vi "SetProtocolState.vi"(9 "state":string) -> ()   [LabVIEW 2018]
uses:
  <vilib>/addons/_JKI.lib/REST Client/classes/REST Client/REST Client.lvclass
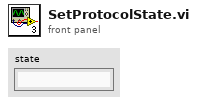
[diagram p1: front panel]
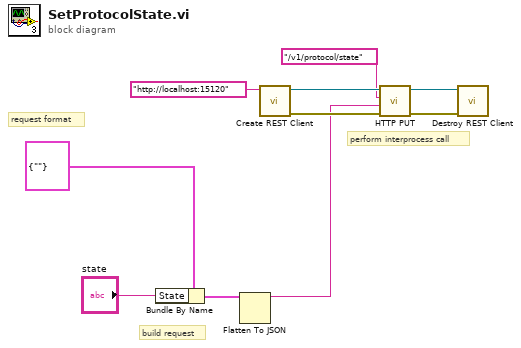
[diagram p0: block diagram]
diagram:
  # "build request"
  # "request format"
  # "perform interprocess call"
  n1 = Bundle By Name(cluster=cluster{"State":string} {"State"=""}, "State"="state") -> (w2:cluster{"State":string})
  n2 = Flatten To JSON(anything=w2) -> (JSON string=w4:string)  [unwired: 2 in, 1 out]
  n3 = call <vilib>:"Create REST Client.vi"("Base URL"="http://localhost:15120") -> ("error out"=w7:errorcluster, "REST Client out"=w9:refnum<class "REST Client.lvclass">)  [unwired: 9 in]
  n4 = call-dynamic "HTTP PUT.vi"("error in (no error)"=w7, "Request body"=w4, "Path"="/v1/protocol/state", "REST Client in"=w9) -> ("error out"=w6:errorcluster, "REST Client out"=w8:refnum<class "REST Client.lvclass">)  [unwired: 2 in, 4 out]
  n5 = call-dynamic "Destroy REST Client.vi"("error in (no error)"=w6, "REST Client in"=w8) -> ()  [unwired: 9 in, 1 out]
